vi "VI Tree.vi"   [LabVIEW 2016, in "Yokogawa WT300 Series.lvlib"]
doc: "This is the instrument driver for the Yokogawa WT300 Series Digital Power Meter. The VI Tree displays all the user-callable VIs of the instrument driver in an organized table."
uses:
  Yokogawa WT300 Series.lvlib
  Data/Read Measurement (Normal).vi
  Data/Low Level/Fetch Measurement (Normal).vi
  Utility/Function/Create Function String (Voltage).vi
panel:
  # "(c) 2013 Yokogawa Meters & Instruments.  All rights reserved."
  # "SEE DIAGRAM\nFOR VI TREE."
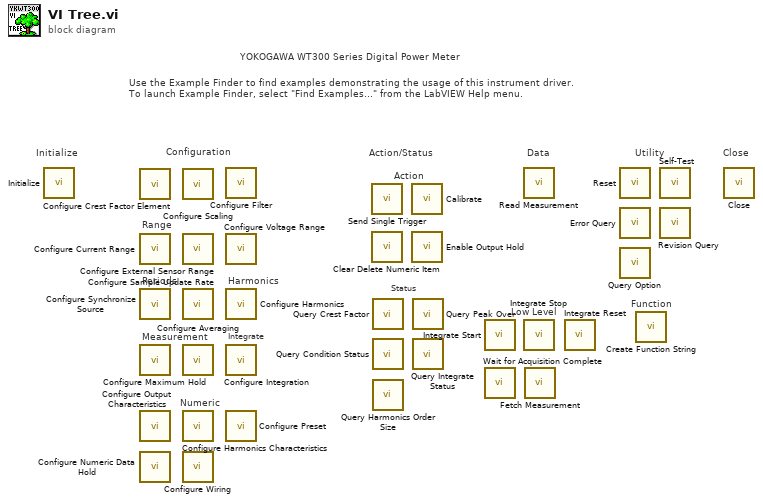
[diagram p0: block diagram]
diagram:
  # "Range"
  # "Low Level"
  # "Numeric"
  # "Status"
  # "Action"
  # "Harmonics"
  # "Integrate"
  # "Function"
  # "Measurement"
  # "Periods"
  # "YOKOGAWA WT300 Series Digital Power Meter"
  # "Use the Example Finder to find examples demonstrating the usage of this instrument driver.\nTo launch Example Finder, select \"Find Examples...\" from the LabVIEW Help menu."
  # "Configuration"
  # "Utility"
  # "Data"
  # "Action/Status"
  # "Close"
  # "Initialize"
  n1 = call "Initialize.vi"() -> ()  [unwired: 9 in, 3 out]
  n2 = call "Configure Crest Factor Element.vi"() -> ()  [unwired: 10 in, 2 out]
  n3 = call "Configure Current Range.vi"() -> ()  [unwired: 14 in, 2 out]
  n4 = call "Configure Synchronize Source.vi"() -> ()  [unwired: 10 in, 2 out]
  n5 = call "Configure Maximum Hold.vi"() -> ()  [unwired: 10 in, 2 out]
  n6 = call "Configure Output Characteristics.vi"() -> ()  [unwired: 10 in, 2 out]
  n7 = call "Configure Numeric Data Hold.vi"() -> ()  [unwired: 10 in, 2 out]
  n8 = call "Configure Scaling.vi"() -> ()  [unwired: 14 in, 2 out]
  n9 = call "Configure External Sensor Range.vi"() -> ()  [unwired: 14 in, 2 out]
  n10 = call "Configure Sample Update Rate.vi"() -> ()  [unwired: 10 in, 2 out]
  n11 = call "Configure Averaging.vi"() -> ()  [unwired: 10 in, 2 out]
  n12 = call "Configure Harmonics Characteristics.vi"() -> ()  [unwired: 10 in, 2 out]
  n13 = call "Configure Wiring.vi"() -> ()  [unwired: 14 in, 2 out]
  n14 = call "Configure Filter.vi"() -> ()  [unwired: 10 in, 2 out]
  n15 = call "Configure Voltage Range.vi"() -> ()  [unwired: 14 in, 2 out]
  n16 = call "Configure Harmonics.vi"() -> ()  [unwired: 14 in, 2 out]
  n17 = call "Configure Integration.vi"() -> ()  [unwired: 14 in, 2 out]
  n18 = call "Configure Preset.vi"() -> ()  [unwired: 10 in, 2 out]
  n19 = call "Send Single Trigger.vi"() -> ()  [unwired: 10 in, 2 out]
  n20 = call "Clear Delete Numeric Item.vi"() -> ()  [unwired: 10 in, 2 out]
  n21 = call "Query Crest Factor.vi"() -> ()  [unwired: 9 in, 3 out]
  n22 = call "Query Condition Status.vi"() -> ()  [unwired: 9 in, 3 out]
  n23 = call "Query Harmonics Order Size.vi"() -> ()  [unwired: 9 in, 3 out]
  n24 = call "Calibrate.vi"() -> ()  [unwired: 9 in, 3 out]
  n25 = call "Enable Output Hold.vi"() -> ()  [unwired: 10 in, 2 out]
  n26 = call "Query Peak Over.vi"() -> ()  [unwired: 8 in, 4 out]
  n27 = call "Query Integrate Status.vi"() -> ()  [unwired: 8 in, 4 out]
  n28 = call "Integrate Start.vi"() -> ()  [unwired: 10 in, 2 out]
  n29 = call "Wait for Acquisition Complete.vi"() -> ()  [unwired: 10 in, 2 out]
  n30 = call-poly "Read Measurement.vi"() -> ()  [unwired: 8 in, 4 out]
  n31 = call "Integrate Stop.vi"() -> ()  [unwired: 10 in, 2 out]
  n32 = call-poly "Fetch Measurement.vi"() -> ()  [unwired: 8 in, 4 out]
  n33 = call "Integrate Reset.vi"() -> ()  [unwired: 10 in, 2 out]
  n34 = call "Reset.vi"() -> ()  [unwired: 10 in, 2 out]
  n35 = call "Error Query.vi"() -> ()  [unwired: 8 in, 4 out]
  n36 = call "Query Option.vi"() -> ()  [unwired: 13 in, 3 out]
  n37 = call-poly "Create Function String.vi"() -> ()  [unwired: 9 in, 3 out]
  n38 = call "Self-Test.vi"() -> ()  [unwired: 8 in, 4 out]
  n39 = call "Revision Query.vi"() -> ()  [unwired: 8 in, 4 out]
  n40 = call "Close.vi"() -> ()  [unwired: 11 in, 1 out]
